vi "启动参数设置.vi"() -> ()   [LabVIEW 2016, in "斯坦道总磷总氮.lvlib"]
uses:
  <vilib>/Utility/miscctls.llb/LVPointTypeDef.ctl
  <vilib>/Utility/config.llb/NI_LVConfig.lvlib
panel:
  in  "启动参数":cluster{"COD":bool, "总氮":bool, "总磷":bool}
  in  "取消":bool
  in  "确认":bool
  # "请选择启动参数"
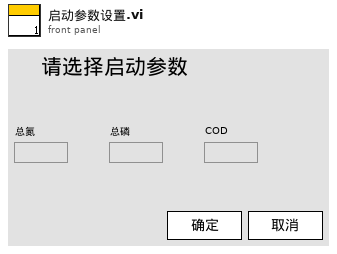
[diagram p1: front panel]
types:
  T1 = typedef "LVPointTypeDef.ctl" = cluster{"Horizontal":i16, "Vertical":i16}
  T2 = typedef "NI_LVConfig.lvlib/Config Data RefNum.ctl" = refnum<k1>
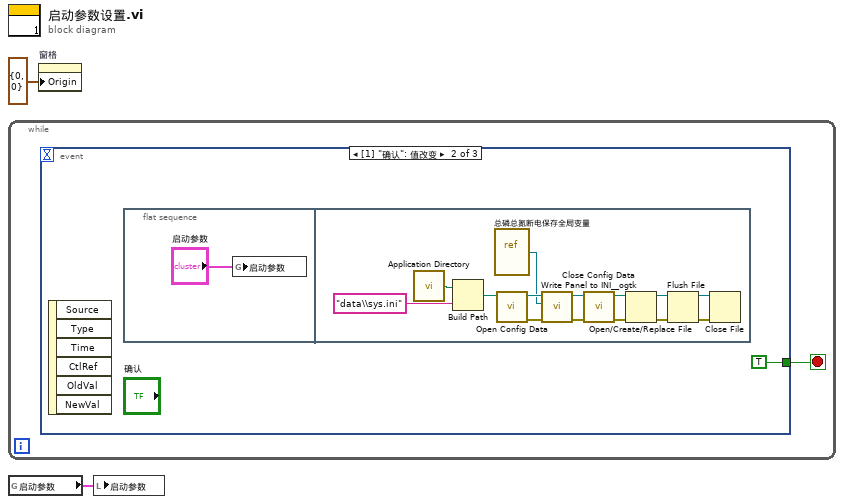
[diagram p0: block diagram]
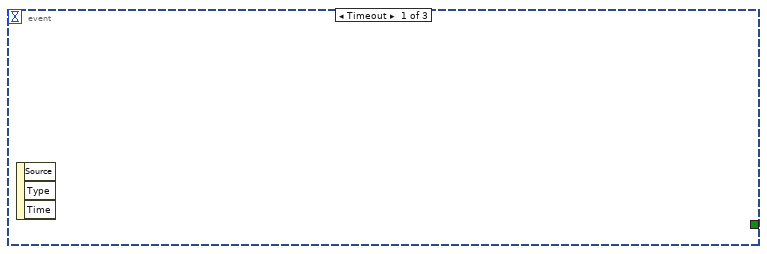
[diagram p2: hidden frame]
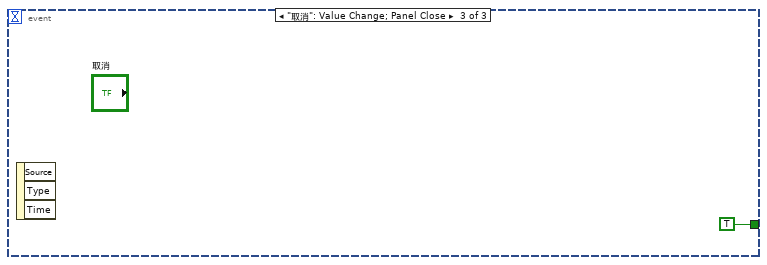
[diagram p3: hidden frame]
diagram:
  n1 = while {
    stop <- w3 stop-if-true
    n2 = event shown="[1] \"确认\": 值改变" {
      selector: _ -> [_ _ _]
      dyn-events: _ -> [_ _ _]
      timeout: _ -> [_ _ _]
      tunnel: [_ TRUE TRUE] -> w3
      event Timeout {
        n3 = event-data() -> ()  [unwired: 1 in, 3 out]
      }
      event "确认": Value Change {
        n4 = event-data() -> ()  [unwired: 1 in, 6 out]
        n5 = flat-sequence {
          frame #0 {
            n6 = global write "总磷总氮断电保存全局变量.vi" "启动参数"("启动参数") -> ()
          }
          frame #1 {
            n7 = call <vilib>:"Application Directory.vi"() -> ("Application Directory"=w19:path)
            n8 = Build Path(base path=w19, name or relative path="data\\sys.ini" ("名称或相对路径")) -> (appended path=w17:path)
            n9 = vi-ref "总磷总氮断电保存全局变量.vi"() -> (w15:refnum<vi>)
            n10 = call <vilib>:"Open Config Data.vi"("configuration file path"=w17) -> ("error out"=w13:errorcluster, "refnum"=w16:T2)  [unwired: 8 in, 1 out]
            n11 = call <userlib>:"Write Panel to INI__ogtk.vi"("error in (no error)"=w13, "VI ref"=w15, "refnum"=w16) -> ("error out"=w12:errorcluster, "refnum out"=w14:T2)  [unwired: 7 in]
            n12 = call <vilib>:"Close Config Data.vi"("error in (no error)"=w12, "refnum"=w14) -> ("error out"=w7:errorcluster, "file path"=w6:path)  [unwired: 8 in]
            n13 = Open/Create/Replace File(file path (use dialog)=w6, error in=w7) -> (refnum out=w10:refnum<file>, error out=w11:errorcluster)  [unwired: 4 in, 1 out]
            n14 = Flush File(refnum=w10, error in=w11) -> (refnum out=w9:refnum<file>, error out=w8:errorcluster)
            n15 = Close File(refnum=w9, error in=w8) -> ()  [unwired: 2 out]
          }
        }
      }
      event "取消": Value Change; Panel Close {
        n16 = event-data() -> ()  [unwired: 1 in, 3 out]
      }
    }
  }
  n17 = global read "总磷总氮断电保存全局变量.vi" "启动参数"() -> (w1:cluster{"COD":bool, "总氮":bool, "总磷":bool})
  n18 = property on="窗格" class="Pane"("Origin"=T1 {"Horizontal"=0, "Vertical"=0} ("原点")) -> ()  [unwired: 2 in, 2 out]
  n19 = local write "启动参数"(w1) -> ()
